vi "DefaultFromIni.vi"(8 "error in (no error)":errorcluster, 11 "AcPwrBase":refnum<class "AcPwrBase.lvclass">) -> (0 "error out":errorcluster, 3 "AcPwrBase":refnum<class "AcPwrBase.lvclass">)   [LabVIEW 2018, in "AcPwrPlugins.lvlib" / "AcPwrBase.lvclass"]
doc: "This VI reads the current configuration stored in the INI file."
uses:
  AcPwrBase.lvclass
  C:/Program Files (x86)/National Instruments/LabVIEW 2018/user.lib/NIST/BaseClasses/BasePlugin_class/BasePlugin.lvclass
  TypeDefs/BaseConfig.ctl
  TypeDefs/Phase.ctl
  TypeDefs/BaseMeasurements.ctl
  TypeDefs/MeasType.ctl
  <userlib>/NIST/BaseClasses/BasePlugin_class/BasePlugin.lvclass/BasePlugin.ctl
  FGen/MemberClasses/FunctionBaseClass/FunctionBase.lvclass
  AcPwrBase.lvclass/AcPwrBase.ctl
  <userlib>/NIST/BaseClasses/BasePlugin_class/Accessors/Read PluginIniFilePath.vi
  <userlib>/NIST/BaseClasses/BasePlugin_class/Accessors/Write PluginIniFilePath.vi
  Accessors/Write BaseConfig.vi
  Accessors/Write FunctionINIFilePath.vi
  Accessors/Write FunctionClass.vi
  Accessors/Write RefreshTime.vi
  <vilib>/Utility/error.llb/Error Cluster From Error Code.vi
  <vilib>/ErrorRing/Error Ring.xnode
  <vilib>/Utility/config.llb/NI_LVConfig.lvlib
  <userlib>/NIST/BaseClasses/Object_class/BaseObject.lvclass
panel:
  out "found?":bool
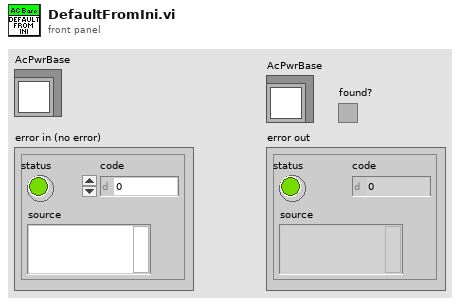
[diagram p1: front panel]
types:
  T1 = typedef "AcPwrPlugins.lvlib/AcPwrBase.lvclass/BaseMeasurements.ctl" = cluster{"Handle":string, "Name":string, "Enabled":bool, "Result":dbl, "MeasType":T2, "btnMeasFetch":bool, "Hold Peak?":bool}[]
  T2 = typedef "AcPwrPlugins.lvlib/AcPwrBase.lvclass/MeasType.ctl" = enum16{"Voltage RMS L-N", "Current RMS", "Frequency", "Voltage DC", "Current DC", "Power Factor", "Current Peak", "Power VA", "Real Power", "Voltage THD", "Voltage EHD", "Voltage OHD", "Current THD", "Current EHD", "Current OHD", "Voltage RMS L-L", "Phase Angle", "Power DC", "Crest Factor"}
  T3 = typedef "AcPwrPlugins.lvlib/AcPwrBase.lvclass/BaseConfig.ctl" = cluster{"Frequency":dbl, "FrequencyRange":dbl[], "Phases":T4[]}
  T4 = typedef "AcPwrPlugins.lvlib/AcPwrBase.lvclass/Phase.ctl" = cluster{"Name":string, "Enabled":bool, "VoltageLevel":dbl, "Handle":string, "VoltageRange":dbl[], "Connected":bool, "CurrentLimit":dbl, "Waveform":string}
  T5 = typedef "NI_LVConfig.lvlib/Config Data RefNum.ctl" = refnum<k1>
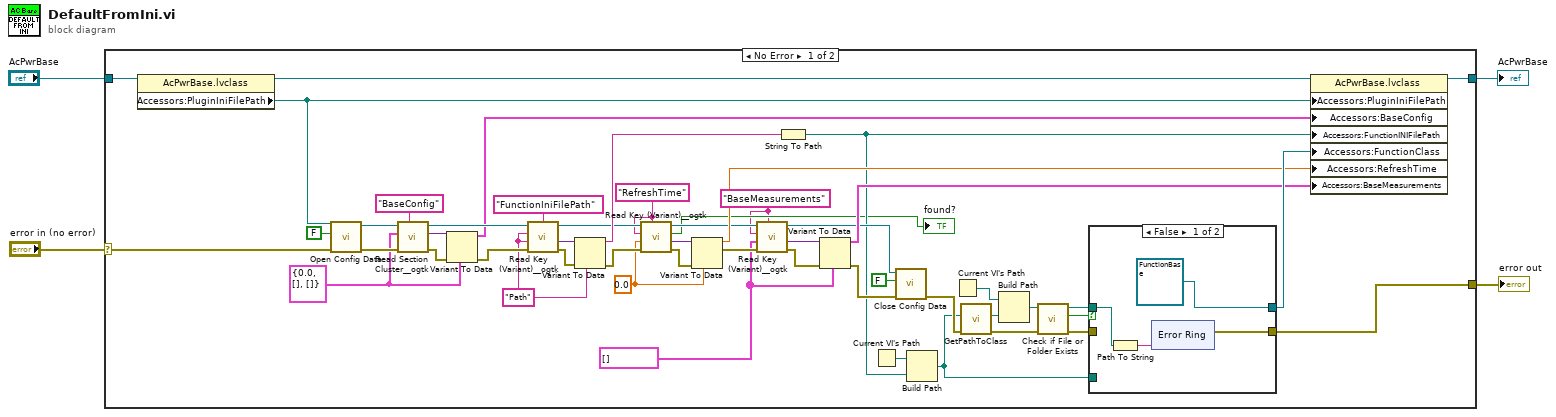
[diagram p0: block diagram]
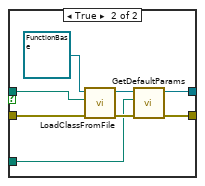
[diagram p2: hidden frame]
diagram:
  n1 = case shown="No Error" "error in (no error)" {
    selector: "error in (no error)" -> [w28 w76]
    tunnel: "AcPwrBase" -> [w30 w75]
    tunnel: [w31 w75] -> w3
    tunnel: [w24 w76] -> w2
    frame No Error {
      w7 = T1 [] ("BaseMeasurements")
      w5 = "BaseMeasurements" ("section")
      w17 = 0.0
      w8 = "RefreshTime" ("section")
      w25 = T3 {"Frequency"=0.0, "FrequencyRange"=[], "Phases"=[]} ("BaseConfig")
      w33 = "Path" ("key (optional)")
      n2 = property class="AcPwrBase.lvclass"(reference=w30) -> (reference out=w29:refnum<class "AcPwrBase.lvclass">, "Accessors:PluginIniFilePath"=w26:path)  [unwired: 1 in, 1 out]
      n3 = call <vilib>:"Open Config Data.vi"("error in (no error)"=w28, "create file if necessary (T)"=FALSE, "configuration file path"=w26) -> ("error out"=w50:errorcluster, "refnum"=w52:T5)  [unwired: 6 in, 1 out]
      n4 = call <userlib>:"Read Section Cluster__ogtk.vi"("section (optional)"="BaseConfig", "error in (no error)"=w50, "Section Formatted Cluster Type"=w25, "refnum"=w52) -> ("error out"=w49:errorcluster, "Section Formatted Cluster"=w54:variant, "dup refnum"=w48:T5)  [unwired: 3 in, 2 out]
      n5 = Variant To Data(error in=w49, type=w25, Variant=w54) -> (data=w23:T3, error out=w47:errorcluster)
      n6 = call <userlib>:"Read Key (Variant)__ogtk.vi"("section"="FunctionIniFilePath", "error in (no error)"=w47, "type"=w33, "key (optional)"=w33, "refnum"=w48) -> ("error out"=w44:errorcluster, "key-value"=w45:variant, "refnum out"=w21:T5)  [unwired: 3 in, 1 out]
      n7 = Variant To Data(error in=w44, type=w33, Variant=w45) -> (data=w35:string, error out=w22:errorcluster)
      n8 = call <userlib>:"Read Key (Variant)__ogtk.vi"("section"=w8, "error in (no error)"=w22, "type"=w17, "key (optional)"=w8, "refnum"=w21) -> ("error out"=w19:errorcluster, "key-value"=w20:variant, "found?"=→"found?":bool, "refnum out"=w15:T5)  [unwired: 3 in]
      n9 = Variant To Data(error in=w19, type=w17, Variant=w20) -> (data=w18:dbl, error out=w16:errorcluster)
      n10 = call <userlib>:"Read Key (Variant)__ogtk.vi"("section"=w5, "error in (no error)"=w16, "type"=w7, "key (optional)"=w5, "refnum"=w15) -> ("error out"=w14:errorcluster, "key-value"=w13:variant, "refnum out"=w10:T5)  [unwired: 3 in, 1 out]
      n11 = String To Path(string=w35) -> (path=w9:path)
      n12 = Variant To Data(error in=w14, type=w7, Variant=w13) -> (data=w11:T1, error out=w12:errorcluster)
      n13 = Current VI's Path() -> (path=w32:path)
      n14 = call <vilib>:"Close Config Data.vi"("error in (no error)"=w12, "write file if changed (T)"=FALSE, "refnum"=w10) -> ("error out"=w36:errorcluster)  [unwired: 7 in, 1 out]
      n15 = Build Path(base path=w32, name or relative path=w9) -> (appended path=w34:path)
      n16 = Current VI's Path() -> (path=w38:path)
      n17 = call <userlib>:"GetPathToClass.vi"("error in (no error)"=w36, "configuration file path"=w34) -> ("error IO"=w41:errorcluster, "PathToClass"=w39:path)  [unwired: 8 in]
      n18 = Build Path(base path=w38, name or relative path=w39) -> (appended path=w37:path)
      n19 = call <vilib>:"Check if File or Folder Exists.vi"("error in (no error)"=w41, "path"=w37) -> ("error out"=w42:errorcluster, "file or folder exists?"=w40:bool, "dup path"=w43:path)  [unwired: 7 in]
      n20 = case shown="False" w40 {
        tunnel: [w58 w69] -> w24
        tunnel: w42 -> [_ w74]
        tunnel: w43 -> [w57 w73]
        tunnel: w34 -> [_ w67]
        tunnel: [refnum<class "FunctionBase.lvclass"> refnum ("Functions.lvlib:FunctionBase.lvclass") w68] -> w27
        frame False {
          n21 = Path To String(path=w57) -> (string=w59:string)
          n22 = xnode "Error Ring"("parameter 0"=w59) -> ("error out"=w58:errorcluster)
        }
        frame True {
          n23 = call-dynamic "LoadClassFromFile.vi"("error in (no error)"=w74, "class path"=w73, "reference in"=refnum<class "FunctionBase.lvclass"> refnum ("Functions.lvlib:FunctionBase.lvclass")) -> ("error out"=w71:errorcluster, "reference out"=w70:refnum<class "FunctionBase.lvclass">)  [unwired: 7 in]
          n24 = call-dynamic "GetDefaultParams.vi"("error in (no error)"=w71, "Path"=w67, "FunctionBase in"=w70) -> ("error out"=w69:errorcluster, "FunctionBase out"=w68:refnum<class "FunctionBase.lvclass">)  [unwired: 7 in]
        }
      }
      n25 = property class="AcPwrBase.lvclass"(reference=w29, "Accessors:PluginIniFilePath"=w26, "Accessors:BaseConfig"=w23, "Accessors:FunctionINIFilePath"=w9, "Accessors:FunctionClass"=w27, "Accessors:RefreshTime"=w18, "Accessors:BaseMeasurements"=w11) -> (reference out=w31:refnum<class "AcPwrBase.lvclass">)  [unwired: 1 in, 1 out]
    }
    frame Error {
    }
  }
  "error out" <- w2
  "AcPwrBase" <- w3
